vi "speaker.vi"() -> ()   [LabVIEW 2019]
panel:
  in  "stop (F)":bool
  in  "error IO":errorcluster
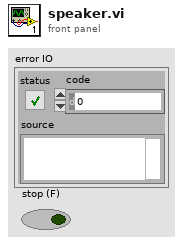
[diagram p1: front panel]
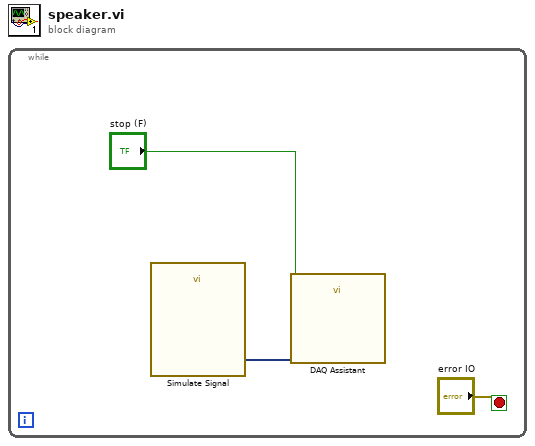
[diagram p0: block diagram]
diagram:
  n1 = while {
    stop <- "error IO" stop-if-true
    n2 = call "Simulate Signal"() -> ("Sine"=w2:dynamicdata)  [unwired: 14 in, 1 out]
    n3 = call "DAQ Assistant"("data"=w2, "stop (F)"="stop (F)") -> ()  [unwired: 15 in, 3 out]
  }
